vi "Finish.vi"   [LabVIEW 2018]
doc: "This VI is called just before exiting. It is expected to close I/O refnum, save collected data, etc."
uses:
  <vilib>/Rock Robotics/WPI/Utilities/WPI_GetSetVariantRefNum.vi
types:
  T1 = typedef "WPI_SwitchDevRef.ctl" = cluster{"DevStatus":errorcluster, "DIO Channel":T2, "CntIndex":T3, "Normally Closed":bool}
  T2 = typedef "FPGA_DIOChannel.ctl" = enum8{"DIO 0", "DIO 1", "DIO 2", "DIO 3", "DIO 4", "DIO 5", "DIO 6", "DIO 7", "DIO 8", "DIO 9", "DIO MXP 0", "DIO MXP 1", "DIO MXP 2", "DIO MXP 3", "DIO MXP 4", "DIO MXP 5", "DIO MXP 6", "DIO MXP 7", "DIO MXP 8", "DIO MXP 9", "DIO MXP 10", "DIO MXP 11", "DIO MXP 12", "DIO MXP 13", "DIO MXP 14", "DIO MXP 15", "SPI Port CS1", "SPI Port CS2", "SPI Port CS3", "SPI Port MISO", "SPI Port MOSI", "Invalid"}
  T3 = typedef "FPGA_CounterCtrSystemIndex.ctl" = enum8{"Ctr 0", "Ctr 1", "Ctr 2", "Ctr 3", "Ctr 4", "Ctr 5", "Ctr 6", "Ctr 7", "Invalid"}
  T4 = typedef "WPI_JoystickDevRef.ctl" = cluster{"Device":T5}
  T5 = typedef "WPI_JoystickDeviceEnum.ctl" = enum16{"USB 0", "USB 1", "USB 2", "USB 3", "USB 4", "USB 5"}
  T6 = typedef "WPI_SolenoidDevRef.ctl" = cluster{"DevStatus":errorcluster, "Pneumatics Control Module":u8, "Forward Solenoid Channel":T7, "Reverse Solenoid Channel":T7}
  T7 = typedef "WPI_SolenoidChannel.ctl" = enum8{"Solenoid 0", "Solenoid 1", "Solenoid 2", "Solenoid 3", "Solenoid 4", "Solenoid 5", "Solenoid 6", "Solenoid 7", "Invalid"}
  T8 = typedef "WPI_CompressorDevRef.ctl" = cluster{"DevStatus":errorcluster, "Pneumatics Control Module":u8}
  T9 = typedef "WPI_MotorControlDeviceRef.ctl" = cluster{"DeviceStatus":errorcluster, "Type":T10, "PWM":cluster{"PWM Channel":T11, "DeadBand":T12}, "CAN":cluster{"Device Number":u8, "SetOutput VI Ref":variant, "GetOutput VI Ref":variant, "Enable VI Ref":variant, "Disable VI Ref":variant, "Data":variant}, "Invert":bool, "DIO PWM":cluster{"PWM \"Enable\" Channel":T11, "DIOChannel":T2, "PWM Rate":dbl}}
  T10 = typedef "WPI_MotorControlType.ctl" = enum16{"PWM", "CAN", "DIO PWM"}
  T11 = typedef "FPGA_DIOPWMChannel.ctl" = enum8{"PWM 0", "PWM 1", "PWM 2", "PWM 3", "PWM 4", "PWM 5", "PWM 6", "PWM 7", "PWM 8", "PWM 9", "PWM MXP 0", "PWM MXP 1", "PWM MXP 2", "PWM MXP 3", "PWM MXP 4", "PWM MXP 5", "PWM MXP 6", "PWM MXP 7", "PWM MXP 8", "PWM MXP 9", "Invalid"}
  T12 = typedef "WPI_PWMDeadband.ctl" = cluster{"Name":string, "maxPositivePwm":i32, "minPositivePwm":i32, "centerPwm":i32, "maxNegativePwm":i32, "minNegativePwm":i32, "angularRange":u16}
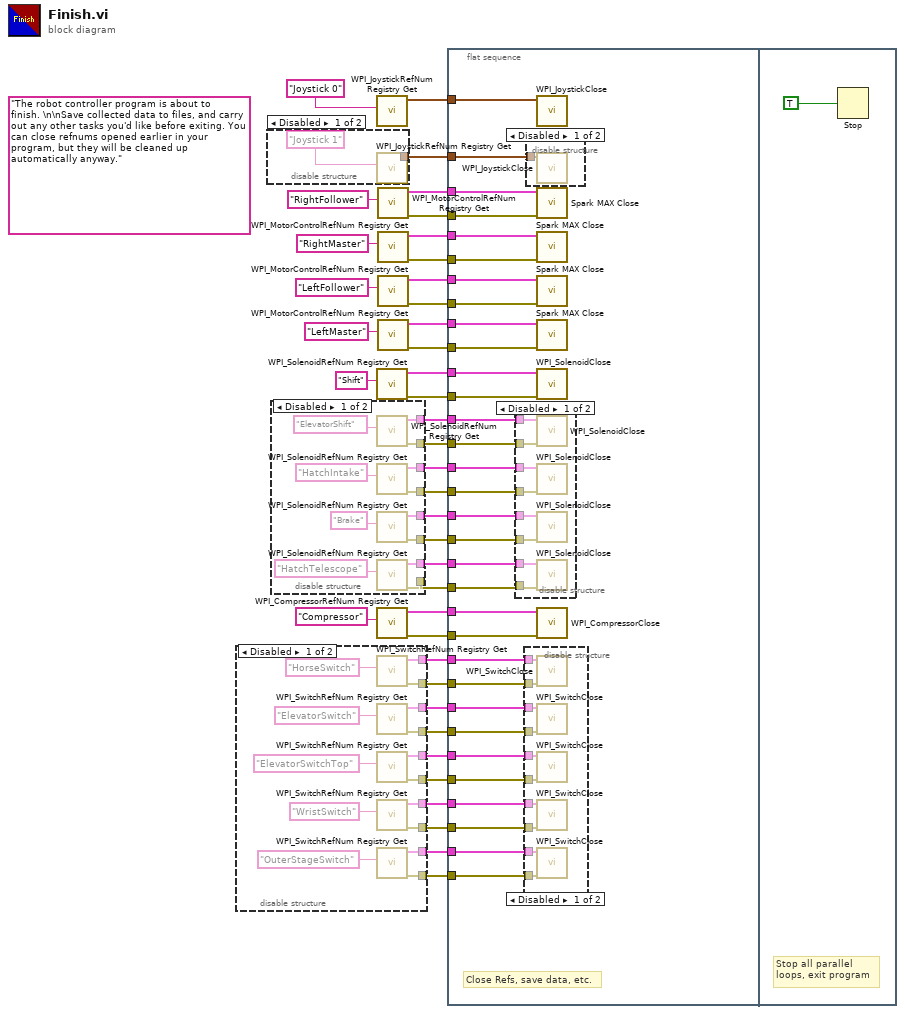
[diagram p0: block diagram]
diagram:
  (unwired) "The robot controller program is about to finish. \n\nSave collected data to files, and carry out any other tasks you'd like before exiting. You can close refnums opened earlier in your program, but they will be cleaned up automatically anyway."
  n1 = disable-structure shown="Disabled" {
    disable-tunnel: [w53 _] -> w14
    disable-tunnel: [w52 _] -> w13
    disable-tunnel: [w51 _] -> w12
    disable-tunnel: [w50 _] -> w11
    disable-tunnel: [w47 _] -> w10
    disable-tunnel: [w46 _] -> w9
    disable-tunnel: [w45 _] -> w8
    disable-tunnel: [w44 _] -> w7
    disable-tunnel: [w41 _] -> w6
    disable-tunnel: [w40 _] -> w5
    frame Disabled {
      n2 = call <vilib>:"WPI_SwitchRefNum Registry Get.vi"("refnum name"="HorseSwitch") -> ("error out"=w52:errorcluster, "SwitchDevRef"=w53:T1)  [unwired: 9 in]
      n3 = call <vilib>:"WPI_SwitchRefNum Registry Get.vi"("refnum name"="ElevatorSwitch") -> ("error out"=w51:errorcluster, "SwitchDevRef"=w50:T1)  [unwired: 9 in]
      n4 = call <vilib>:"WPI_SwitchRefNum Registry Get.vi"("refnum name"="ElevatorSwitchTop") -> ("error out"=w46:errorcluster, "SwitchDevRef"=w47:T1)  [unwired: 9 in]
      n5 = call <vilib>:"WPI_SwitchRefNum Registry Get.vi"("refnum name"="WristSwitch") -> ("error out"=w45:errorcluster, "SwitchDevRef"=w44:T1)  [unwired: 9 in]
      n6 = call <vilib>:"WPI_SwitchRefNum Registry Get.vi"("refnum name"="OuterStageSwitch") -> ("error out"=w40:errorcluster, "SwitchDevRef"=w41:T1)  [unwired: 9 in]
    }
    frame Enabled {
    }
  }
  n7 = disable-structure shown="Disabled" {
    disable-tunnel: [w56 _] -> w15
    frame Disabled {
      n8 = call <vilib>:"WPI_JoystickRefNum Registry Get.vi"("refnum name"="Joystick 1") -> ("JoystickDevRef"=w56:T4)  [unwired: 1 in, 9 out]
    }
    frame Enabled {
    }
  }
  n9 = disable-structure shown="Disabled" {
    disable-tunnel: [w68 _] -> w22
    disable-tunnel: [w67 _] -> w21
    disable-tunnel: [w64 _] -> w20
    disable-tunnel: [w63 _] -> w19
    disable-tunnel: [w61 _] -> w4
    disable-tunnel: [w60 _] -> w3
    disable-tunnel: [w59 _] -> w2
    disable-tunnel: [w58 _] -> w1
    frame Disabled {
      n10 = call <vilib>:"WPI_SolenoidRefNum Registry Get.vi"("refnum name"="ElevatorShift") -> ("error out"=w64:errorcluster, "SolenoidDevRef"=w63:T6)  [unwired: 9 in]
      n11 = call <vilib>:"WPI_SolenoidRefNum Registry Get.vi"("refnum name"="HatchIntake") -> ("error out"=w67:errorcluster, "SolenoidDevRef"=w68:T6)  [unwired: 9 in]
      n12 = call <vilib>:"WPI_SolenoidRefNum Registry Get.vi"("refnum name"="Brake") -> ("error out"=w61:errorcluster, "SolenoidDevRef"=w60:T6)  [unwired: 9 in]
      n13 = call <vilib>:"WPI_SolenoidRefNum Registry Get.vi"("refnum name"="HatchTelescope") -> ("error out"=w58:errorcluster, "SolenoidDevRef"=w59:T6)  [unwired: 9 in]
    }
    frame Enabled {
    }
  }
  n14 = call <vilib>:"WPI_JoystickRefNum Registry Get.vi"("refnum name"="Joystick 0") -> ("JoystickDevRef"=w38:T4)  [unwired: 1 in, 9 out]
  n15 = call <vilib>:"WPI_SolenoidRefNum Registry Get.vi"("refnum name"="Shift") -> ("error out"=w24:errorcluster, "SolenoidDevRef"=w25:T6)  [unwired: 9 in]
  n16 = call <vilib>:"WPI_CompressorRefNum Registry Get.vi"("refnum name"="Compressor") -> ("error out"=w17:errorcluster, "CompressorDevRef"=w18:T8)  [unwired: 9 in]
  n17 = call <vilib>:"WPI_MotorControlRefNum Registry Get.vi"("refnum name"="RightFollower") -> ("error out"=w36:errorcluster, "MotorControlDevRef"=w37:T9)  [unwired: 9 in]
  n18 = call <vilib>:"WPI_MotorControlRefNum Registry Get.vi"("refnum name"="RightMaster") -> ("error out"=w33:errorcluster, "MotorControlDevRef"=w32:T9)  [unwired: 9 in]
  n19 = call <vilib>:"WPI_MotorControlRefNum Registry Get.vi"("refnum name"="LeftFollower") -> ("error out"=w27:errorcluster, "MotorControlDevRef"=w26:T9)  [unwired: 9 in]
  n20 = call <vilib>:"WPI_MotorControlRefNum Registry Get.vi"("refnum name"="LeftMaster") -> ("error out"=w30:errorcluster, "MotorControlDevRef"=w31:T9)  [unwired: 9 in]
  n21 = flat-sequence {
    tunnel: w38 -> [w100]
    tunnel: w37 -> [w99]
    tunnel: w36 -> [w98]
    tunnel: w32 -> [w96]
    tunnel: w33 -> [w97]
    tunnel: w26 -> [w92]
    tunnel: w27 -> [w93]
    tunnel: w31 -> [w95]
    tunnel: w30 -> [w94]
    tunnel: w25 -> [w91]
    tunnel: w24 -> [w90]
    tunnel: w19 -> [w86]
    tunnel: w20 -> [w87]
    tunnel: w22 -> [w89]
    tunnel: w21 -> [w88]
    tunnel: w18 -> [w85]
    tunnel: w17 -> [w84]
    tunnel: w15 -> [w83]
    tunnel: w14 -> [w82]
    tunnel: w13 -> [w81]
    tunnel: w11 -> [w79]
    tunnel: w12 -> [w80]
    tunnel: w10 -> [w78]
    tunnel: w9 -> [w77]
    tunnel: w7 -> [w75]
    tunnel: w8 -> [w76]
    tunnel: w6 -> [w74]
    tunnel: w5 -> [w73]
    tunnel: w3 -> [w71]
    tunnel: w4 -> [w72]
    tunnel: w2 -> [w70]
    tunnel: w1 -> [w69]
    frame #0 {
      # "Close Refs, save data, etc."
      n22 = disable-structure shown="Disabled" {
        disable-tunnel: w89 -> [w119 _]
        disable-tunnel: w88 -> [w118 _]
        disable-tunnel: w87 -> [w117 _]
        disable-tunnel: w86 -> [w116 _]
        disable-tunnel: w72 -> [w115 _]
        disable-tunnel: w71 -> [w114 _]
        disable-tunnel: w70 -> [w113 _]
        disable-tunnel: w69 -> [w112 _]
        frame Disabled {
          n23 = call <vilib>:"WPI_SolenoidClose.vi"("error in (no error)"=w117, "SolenoidDevRef"=w116) -> ()  [unwired: 9 in, 1 out]
          n24 = call <vilib>:"WPI_SolenoidClose.vi"("error in (no error)"=w118, "SolenoidDevRef"=w119) -> ()  [unwired: 9 in, 1 out]
          n25 = call <vilib>:"WPI_SolenoidClose.vi"("error in (no error)"=w115, "SolenoidDevRef"=w114) -> ()  [unwired: 9 in, 1 out]
          n26 = call <vilib>:"WPI_SolenoidClose.vi"("error in (no error)"=w112, "SolenoidDevRef"=w113) -> ()  [unwired: 9 in, 1 out]
        }
        frame Enabled {
        }
      }
      n27 = disable-structure shown="Disabled" {
        disable-tunnel: w82 -> [w111 _]
        disable-tunnel: w81 -> [w110 _]
        disable-tunnel: w80 -> [w109 _]
        disable-tunnel: w79 -> [w108 _]
        disable-tunnel: w78 -> [w107 _]
        disable-tunnel: w77 -> [w106 _]
        disable-tunnel: w76 -> [w105 _]
        disable-tunnel: w75 -> [w104 _]
        disable-tunnel: w74 -> [w103 _]
        disable-tunnel: w73 -> [w102 _]
        frame Disabled {
          n28 = call <vilib>:"WPI_SwitchClose.vi"("error in (no error)"=w110, "SwitchDevRef"=w111) -> ()  [unwired: 9 in, 1 out]
          n29 = call <vilib>:"WPI_SwitchClose.vi"("error in (no error)"=w109, "SwitchDevRef"=w108) -> ()  [unwired: 9 in, 1 out]
          n30 = call <vilib>:"WPI_SwitchClose.vi"("error in (no error)"=w106, "SwitchDevRef"=w107) -> ()  [unwired: 9 in, 1 out]
          n31 = call <vilib>:"WPI_SwitchClose.vi"("error in (no error)"=w105, "SwitchDevRef"=w104) -> ()  [unwired: 9 in, 1 out]
          n32 = call <vilib>:"WPI_SwitchClose.vi"("error in (no error)"=w102, "SwitchDevRef"=w103) -> ()  [unwired: 9 in, 1 out]
        }
        frame Enabled {
        }
      }
      n33 = disable-structure shown="Disabled" {
        disable-tunnel: w83 -> [w101 _]
        frame Disabled {
          n34 = call <vilib>:"WPI_JoystickClose.vi"("JoystickDevRef"=w101) -> ()  [unwired: 11 out]
        }
        frame Enabled {
        }
      }
      n35 = call <vilib>:"WPI_JoystickClose.vi"("JoystickDevRef"=w100) -> ()  [unwired: 11 out]
      n36 = call <vilib>:"Spark MAX Close.vi"("error in"=w98, "MotorControlDeviceRef"=w99) -> ()  [unwired: 9 in, 1 out]
      n37 = call <vilib>:"Spark MAX Close.vi"("error in"=w97, "MotorControlDeviceRef"=w96) -> ()  [unwired: 9 in, 1 out]
      n38 = call <vilib>:"Spark MAX Close.vi"("error in"=w93, "MotorControlDeviceRef"=w92) -> ()  [unwired: 9 in, 1 out]
      n39 = call <vilib>:"Spark MAX Close.vi"("error in"=w94, "MotorControlDeviceRef"=w95) -> ()  [unwired: 9 in, 1 out]
      n40 = call <vilib>:"WPI_SolenoidClose.vi"("error in (no error)"=w90, "SolenoidDevRef"=w91) -> ()  [unwired: 9 in, 1 out]
      n41 = call <vilib>:"WPI_CompressorClose.vi"("error in (no error)"=w84, "CompressorDevRef"=w85) -> ()  [unwired: 9 in, 1 out]
    }
    frame #1 {
      # "Stop all parallel\nloops, exit program"
      n42 = Stop(stop? (T)=TRUE ("Quit")) -> ()
    }
  }
